vi "getecefdcmref.vi"(0 "map name":T1(ring)) -> (4 "XYZ":dbl[](array[numeric]), 6 "dcm":dbl[][](array[numeric]), 8 "lat":dbl, 10 "lon":dbl, 15 "height":dbl)   [LabVIEW 2015]
panel:
  out "sin(phi)":dbl
  out "cos(phi)":dbl
  out "sin(lam)":dbl
  out "cos(lam)":dbl
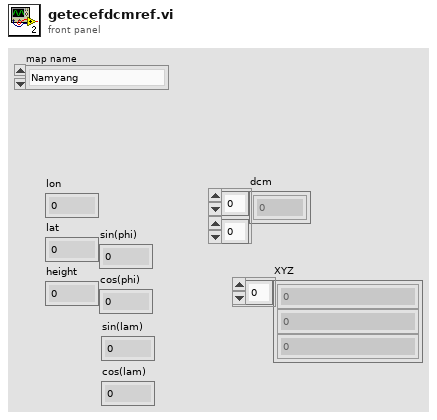
[diagram p1: front panel]
types:
  T1 = enum32{"Namyang", "Hyundai", "KAIST", "Ajou", "Munji", "Airforce", "Car", "KATRI", "Samsung", "Coex", "Gwangnaru", "Inje", "sinjin", "NAVER"}
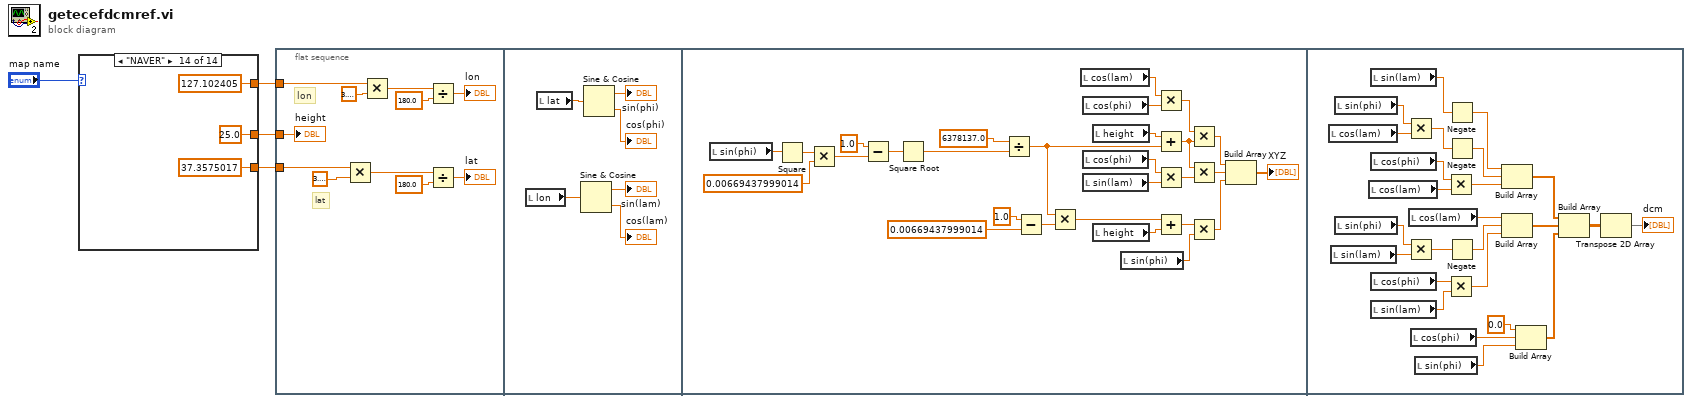
[diagram p0: block diagram]
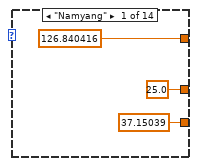
[diagram p2: hidden frame]
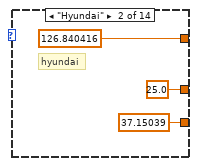
[diagram p3: hidden frame]
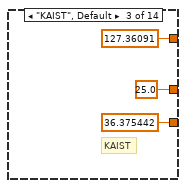
[diagram p4: hidden frame]
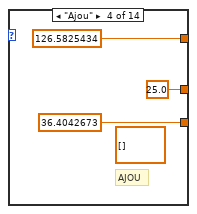
[diagram p5: hidden frame]
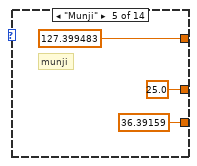
[diagram p6: hidden frame]
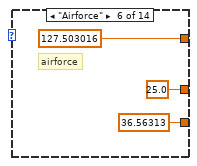
[diagram p7: hidden frame]
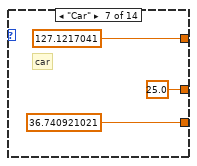
[diagram p8: hidden frame]
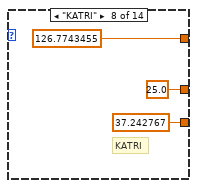
[diagram p9: hidden frame]
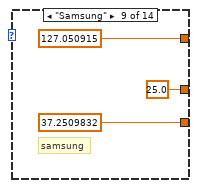
[diagram p10: hidden frame]
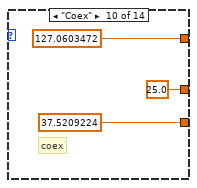
[diagram p11: hidden frame]
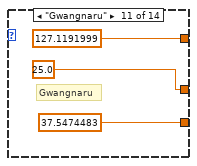
[diagram p12: hidden frame]
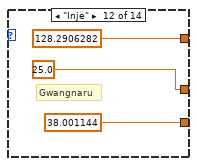
[diagram p13: hidden frame]
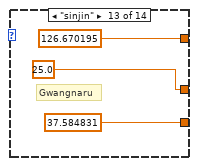
[diagram p14: hidden frame]
diagram:
  n1 = case shown="\"NAVER\"" "map name" {
    tunnel: [37.15039 ("lat0") 37.15039 ("lat0") 36.375442 ("lat0") 36.4042673 ("lat0") 36.39159 ("lat0") 36.56313 ("lat0") 36.740921021 ("lat0") 37.242767 ("lat0") 37.2509832 ("lat0") 37.5209224 ("lat0") 37.5474483 ("lat0") 38.001144 ("lat0") 37.584831 ("lat0") 37.3575017 ("lat0")] -> w3
    tunnel: [126.840416 ("lon0") 126.840416 ("lon0") 127.36091 ("lon0") 126.5825434 ("lon0") 127.399483 ("lon0") 127.503016 ("lon0") 127.1217041 ("lon0") 126.7743455 ("lon0") 127.050915 ("lon0") 127.0603472 ("lon0") 127.1191999 ("lon0") 128.2906282 ("lon0") 126.670195 ("lon0") 127.102405 ("lon0")] -> w4
    tunnel: [25.0 ("height0") 25.0 ("height0") 25.0 ("height0") 25.0 ("height0") 25.0 ("height0") 25.0 ("height0") 25.0 ("height0") 25.0 ("height0") 25.0 ("height0") 25.0 ("height0") 25.0 ("height0") 25.0 ("height0") 25.0 ("height0") 25.0 ("height0")] -> w2
    frame "Namyang" {
    }
    frame "Hyundai" {
      # "hyundai"
    }
    frame "KAIST", Default {
      # "KAIST"
    }
    frame "Ajou" {
      (unwired) dbl[][] [] ("array")
      # "AJOU"
    }
    frame "Munji" {
      # "munji"
    }
    frame "Airforce" {
      # "airforce"
    }
    frame "Car" {
      # "car"
    }
    frame "KATRI" {
      # "KATRI"
    }
    frame "Samsung" {
      # "samsung"
    }
    frame "Coex" {
      # "coex"
    }
    frame "Gwangnaru" {
      # "Gwangnaru"
    }
    frame "Inje" {
      # "Gwangnaru"
    }
    frame "sinjin" {
      # "Gwangnaru"
    }
    frame "NAVER" {
    }
  }
  n2 = flat-sequence {
    tunnel: w4 -> [w49]
    tunnel: w3 -> [w48]
    tunnel: w2 -> [w47]
    frame #0 {
      # "lon"
      # "lat"
      n3 = Multiply(x=w48, y=3.141592653589793) -> (x*y=w56:dbl)
      n4 = Multiply(x=w49, y=3.141592653589793) -> (x*y=w53:dbl)
      n5 = Divide(x=w53, y=180.0) -> (x/y=→"lon":dbl)
      n6 = Divide(x=w56, y=180.0) -> (x/y=→"lat":dbl)
      "height" <- w47
    }
    frame #1 {
      n7 = local read "lon"() -> (w58:dbl)
      n8 = local read "lat"() -> (w63:dbl)
      n9 = Sine & Cosine(0:w58) -> (1:→"sin(lam)":dbl, 2:→"cos(lam)":dbl)
      n10 = Sine & Cosine(0:w63) -> (1:→"sin(phi)":dbl, 2:→"cos(phi)":dbl)
    }
    frame #2 {
      n11 = local read "sin(phi)"() -> (w75:dbl)
      n12 = Square(x=w75) -> (x^2=w90:dbl)
      n13 = Multiply(x=w90, y=0.00669437999014) -> (x*y=w89:dbl)
      n14 = Subtract(x=1.0, y=w89) -> (x-y=w85:dbl)
      n15 = Square Root(x=w85) -> (sqrt(x)=w87:dbl)
      n16 = Divide(x=6378137.0, y=w87) -> (x/y=w77:dbl)
      n17 = Subtract(x=1.0, y=0.00669437999014) -> (x-y=w76:dbl)
      n18 = Multiply(x=w77, y=w76) -> (x*y=w82:dbl)
      n19 = local read "cos(lam)"() -> (w70:dbl)
      n20 = local read "cos(phi)"() -> (w67:dbl)
      n21 = local read "cos(phi)"() -> (w71:dbl)
      n22 = local read "sin(lam)"() -> (w69:dbl)
      n23 = local read "height"() -> (w74:dbl)
      n24 = local read "height"() -> (w73:dbl)
      n25 = local read "sin(phi)"() -> (w72:dbl)
      n26 = Multiply(x=w70, y=w67) -> (x*y=w68:dbl)
      n27 = Add(x=w74, y=w77) -> (x+y=w66:dbl)
      n28 = Multiply(x=w71, y=w69) -> (x*y=w65:dbl)
      n29 = Add(x=w82, y=w73) -> (x+y=w78:dbl)
      n30 = Multiply(x=w68, y=w66) -> (x*y=w81:dbl)
      n31 = Multiply(x=w66, y=w65) -> (x*y=w80:dbl)
      n32 = Multiply(x=w78, y=w72) -> (x*y=w79:dbl)
      n33 = Build Array(w81, w80, w79) -> (→"XYZ":dbl[])
    }
    frame #3 {
      n34 = local read "cos(lam)"() -> (w113:dbl)
      n35 = local read "sin(lam)"() -> (w102:dbl)
      n36 = local read "sin(phi)"() -> (w114:dbl)
      n37 = local read "sin(phi)"() -> (w101:dbl)
      n38 = local read "cos(lam)"() -> (w110:dbl)
      n39 = local read "sin(lam)"() -> (w116:dbl)
      n40 = local read "cos(phi)"() -> (w109:dbl)
      n41 = local read "cos(phi)"() -> (w106:dbl)
      n42 = local read "sin(lam)"() -> (w105:dbl)
      n43 = Multiply(x=w114, y=w113) -> (x*y=w112:dbl)
      n44 = Multiply(x=w101, y=w102) -> (x*y=w103:dbl)
      n45 = local read "cos(lam)"() -> (w100:dbl)
      n46 = local read "cos(phi)"() -> (w98:dbl)
      n47 = local read "sin(phi)"() -> (w97:dbl)
      n48 = Multiply(x=w109, y=w110) -> (x*y=w108:dbl)
      n49 = Multiply(x=w106, y=w105) -> (x*y=w107:dbl)
      n50 = Negate(x=w116) -> (-x=w115:dbl)
      n51 = Negate(x=w112) -> (-x=w111:dbl)
      n52 = Negate(x=w103) -> (-x=w104:dbl)
      n53 = Build Array(w115, w111, w108) -> (w96:dbl[])
      n54 = Build Array(w100, w104, w107) -> (w95:dbl[])
      n55 = Build Array(0.0 ("element"), w98, w97) -> (w94:dbl[])
      n56 = Build Array(w96, w95, w94) -> (w93:dbl[][])
      n57 = Transpose 2D Array(2D array=w93) -> (transposed array=→"dcm":dbl[][])
    }
  }
